vi "_2062021.vi"() -> ()   [LabVIEW 2020]
panel:
  in  "Stop Button":bool
  in  "LOAD":bool
  in  "SAVE":bool
  in  "Tremolo Enable":bool
  in  "Number of samples":i32=50000
  out "Tremolo Graph":dynamicdata(graph)
  in  "Tremelo Frequency":dbl(slide) scale=0.0..10.0
  in  "offset":dbl(slide) scale=0.0..10.0
  in  "Amplitude":dbl(slide) scale=0.0..10.0
  out "EQ Cluster":T1 {"Treble" scale=0.0..10.0; "Mid4" scale=0.0..10.0; "Mid3" scale=0.0..10.0; "Mid2" scale=0.0..10.0; "Mid1" scale=0.0..10.0; "Bass" scale=0.0..10.0}
  out "Output Graph":dynamicdata(graph)
  in  "Panning Enable":bool
  out "Equalizer Graph":dynamicdata(graph)
  in  "Enum":T2(ring)
  in  "Custom cluster":T1 {"Treble" scale=0.0..10.0; "Mid4" scale=0.0..10.0; "Mid3" scale=0.0..10.0; "Mid2" scale=0.0..10.0; "Mid1" scale=0.0..10.0; "Bass" scale=0.0..10.0}
  in  "EQ Enable":bool
  in  "Sampling rate":dbl=100000.0
  out "Panning Graph":dynamicdata(graph)
  in  "Panning Knob":dbl(knob) scale=-2.0..2.0
  in  "STOP":bool
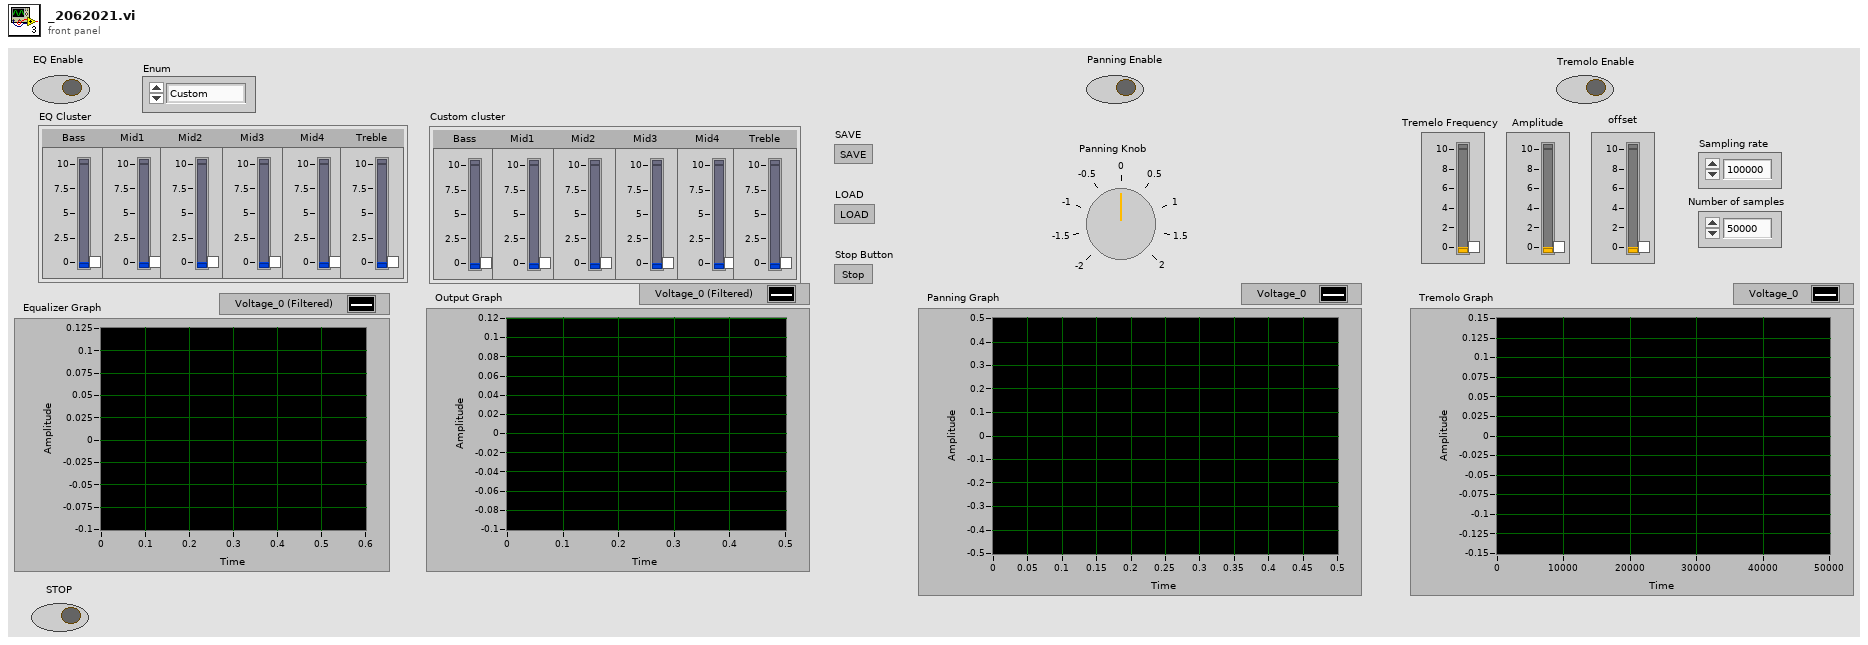
[diagram p1: front panel]
types:
  T1 = cluster{"Bass":dbl, "Mid1":dbl, "Mid2":dbl, "Mid3":dbl, "Mid4":dbl, "Treble":dbl}
  T2 = enum16{"Custom", "Flat", "Treble Boost", "Base Boost"}
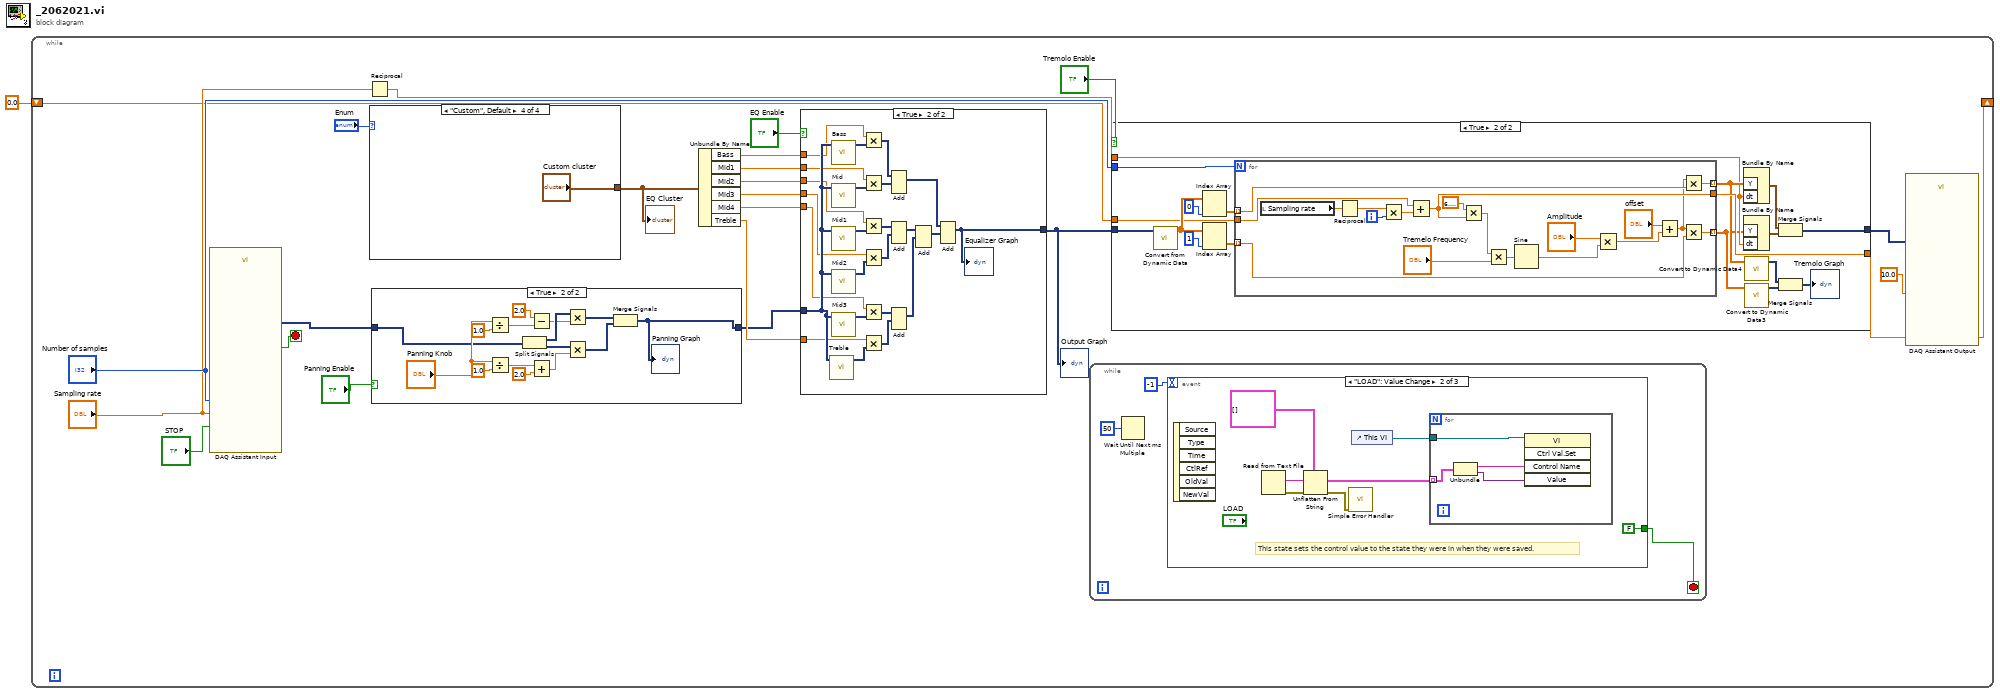
[diagram p0: block diagram]
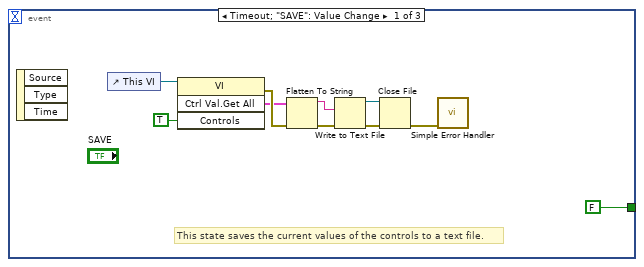
[diagram p2: hidden frame]
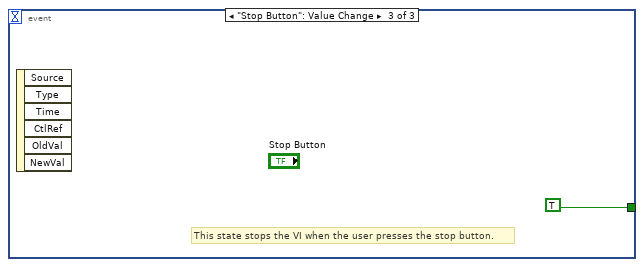
[diagram p3: hidden frame]
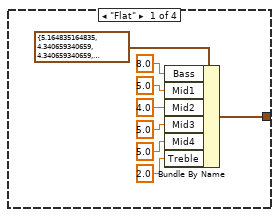
[diagram p6: hidden frame]
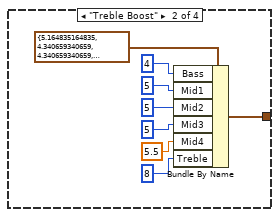
[diagram p7: hidden frame]
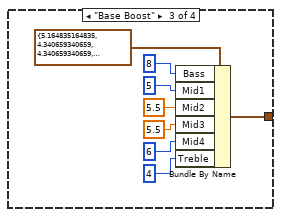
[diagram p8: hidden frame]
diagram:
  n1 = while {
    shift-right: [w10] -> _
    shift-left: 0.0 -> [w3]
    stop <- w23 stop-if-true
    n2 = call "DAQ Assistant Input"("rate"="Sampling rate", "number of samples"="Number of samples", "stop (F)"="STOP") -> ("data"=w15:dynamicdata, "stopped"=w23:bool)  [unwired: 13 in, 2 out]
    n3 = Reciprocal(x="Sampling rate") -> (1/x=w8:dbl)
    n4 = case shown="\"Custom\", Default" "Enum" {
      tunnel: [w105 w113 w121 "Custom cluster"] -> w11
      frame "Flat" {
        n5 = Bundle By Name(cluster=T1 {"Bass"=5.164835164835, "Mid1"=4.340659340659, "Mid2"=4.340659340659, "Mid3"=4.67032967033, "Mid4"=4.450549450549, "Treble"=5.3846153846149996} ("output cluster"), "Bass"=8.0, "Mid1"=5.0 ("Bass"), "Mid2"=4.0 ("Bass"), "Mid3"=5.0 ("Bass"), "Mid4"=5.0 ("Bass"), "Treble"=2.0 ("Bass")) -> (w105:T1)
      }
      frame "Treble Boost" {
        n6 = Bundle By Name(cluster=T1 {"Bass"=5.164835164835, "Mid1"=4.340659340659, "Mid2"=4.340659340659, "Mid3"=4.67032967033, "Mid4"=4.450549450549, "Treble"=5.3846153846149996} ("output cluster"), "Bass"=4, "Mid1"=5, "Mid2"=5, "Mid3"=5, "Mid4"=5.5, "Treble"=8) -> (w113:T1)
      }
      frame "Base Boost" {
        n7 = Bundle By Name(cluster=T1 {"Bass"=5.164835164835, "Mid1"=4.340659340659, "Mid2"=4.340659340659, "Mid3"=4.67032967033, "Mid4"=4.450549450549, "Treble"=5.3846153846149996} ("input cluster"), "Bass"=8, "Mid1"=5, "Mid2"=5.5, "Mid3"=5.5, "Mid4"=6, "Treble"=4) -> (w121:T1)
      }
      frame "Custom", Default {
      }
    }
    "EQ Cluster" <- w11
    n8 = case shown="True" "Panning Enable" {
      tunnel: w15 -> [w89 w91]
      tunnel: [w89 w90] -> w14
      frame False {
      }
      frame True {
        n9 = Divide(x="Panning Knob", y=1.0) -> (x/y=w102:dbl)
        n10 = Divide(x="Panning Knob", y=1.0) -> (x/y=w95:dbl)
        n11 = Split Signals(w91) -> (w104:dynamicdata, w94:dynamicdata)  [unwired: 2 in]
        n12 = Subtract(x=2.0, y=w102) -> (x-y=w100:dbl)
        n13 = Add(x=w95, y=2.0 ("x")) -> (x+y=w97:dbl)
        n14 = Multiply(x=w104, y=w100) -> (x*y=w93:dynamicdata)
        n15 = Multiply(x=w94, y=w97) -> (x*y=w92:dynamicdata)
        n16 = Merge Signals(w93, w92) -> (w90:dynamicdata)
        "Panning Graph" <- w90
      }
    }
    n17 = Unbundle By Name(w11) -> ("Bass"=w22:dbl, "Mid1"=w21:dbl, "Mid2"=w20:dbl, "Mid3"=w19:dbl, "Mid4"=w18:dbl, "Treble"=w17:dbl)
    n18 = case shown="True" "EQ Enable" {
      tunnel: w14 -> [w130 w154]
      tunnel: w22 -> [_ w147]
      tunnel: w21 -> [_ w146]
      tunnel: w20 -> [_ w145]
      tunnel: w19 -> [_ w144]
      tunnel: w18 -> [_ w143]
      tunnel: w17 -> [_ w142]
      tunnel: [w130 w132] -> w9
      frame False {
      }
      frame True {
        n19 = call "Treble"("Signal"=w154) -> ("Filtered Signal"=w148:dynamicdata)  [unwired: 9 in, 1 out]
        n20 = call "Bass"("Signal"=w154) -> ("Filtered Signal"=w153:dynamicdata)  [unwired: 9 in, 1 out]
        n21 = call "Mid"("Signal"=w154) -> ("Filtered Signal"=w152:dynamicdata)  [unwired: 9 in, 1 out]
        n22 = call "Mid1"("Signal"=w154) -> ("Filtered Signal"=w151:dynamicdata)  [unwired: 9 in, 1 out]
        n23 = call "Mid2"("Signal"=w154) -> ("Filtered Signal"=w150:dynamicdata)  [unwired: 9 in, 1 out]
        n24 = call "Mid3"("Signal"=w154) -> ("Filtered Signal"=w149:dynamicdata)  [unwired: 9 in, 1 out]
        n25 = Multiply(x=w147, y=w153) -> (x*y=w141:dynamicdata)
        n26 = Multiply(x=w146, y=w152) -> (x*y=w140:dynamicdata)
        n27 = Multiply(x=w145, y=w151) -> (x*y=w139:dynamicdata)
        n28 = Multiply(x=w144, y=w150) -> (x*y=w138:dynamicdata)
        n29 = Multiply(x=w143, y=w149) -> (x*y=w137:dynamicdata)
        n30 = Multiply(x=w142, y=w148) -> (x*y=w136:dynamicdata)
        n31 = Add(1:w140, 2:w141) -> (0:w133:dynamicdata)  [unwired: 1 in, 1 out]
        n32 = Add(1:w138, 2:w139) -> (0:w135:dynamicdata)  [unwired: 1 in, 1 out]
        n33 = Add(1:w136, 2:w137) -> (0:w131:dynamicdata)  [unwired: 1 in, 1 out]
        n34 = Add(1:w131, 2:w135) -> (0:w134:dynamicdata)  [unwired: 1 in, 1 out]
        n35 = Add(1:w134, 2:w133) -> (0:w132:dynamicdata)  [unwired: 1 in, 1 out]
        "Equalizer Graph" <- w132
      }
    }
    "Output Graph" <- w9
    n36 = while {
      stop <- w27 stop-if-true
      n37 = Wait Until Next ms Multiple(millisecond multiple=u32 50) -> ()  [unwired: 1 out]
      n38 = event shown="[1] \"LOAD\": Value Change" {
        selector: _ -> [_ _ _]
        dyn-events: _ -> [_ _ _]
        timeout: -1 -> [_ _ _]
        tunnel: [FALSE FALSE TRUE] -> w27
        event Timeout; "SAVE": Value Change {
          # "This state saves the current values of the controls to a text file."
          n39 = event-data() -> ()  [unwired: 1 in, 3 out]
          n40 = control-ref of="This VI"() -> (w37:refnum<vi>)
          n41 = invoke class="VI" method="Ctrl Val.Get All"(reference=w37, "Controls"=TRUE) -> (error out=w33:errorcluster, "Get All Control Values Variant"=w32:cluster{"Name":string, "Variant Data":variant}[])  [unwired: 2 in, 2 out]
          n42 = Flatten To String(anything=w32, error in (no error)=w33) -> (data string=w34:string, error out=w35:errorcluster)  [unwired: 2 in, 1 out]
          n43 = Write to Text File(text=w34, error in=w35) -> (refnum out=w30:refnum<file>, error out=w31:errorcluster)  [unwired: 2 in, 1 out]
          n44 = Close File(refnum=w30, error in=w31) -> (error out=w29:errorcluster)  [unwired: 1 out]
          n45 = call <vilib>:"Simple Error Handler.vi"("error in (no error)"=w29) -> ()  [unwired: 4 in, 5 out]
        }
        event "LOAD": Value Change {
          # "This state sets the control value to the state they were in when they were saved."
          n46 = event-data() -> ()  [unwired: 1 in, 6 out]
          n47 = Read from Text File() -> (text=w42:string, error out=w43:errorcluster)  [unwired: 4 in, 2 out]
          n48 = Unflatten From String(type=cluster{string, variant}[] [], binary string=w42, error in (no error)=w43) -> (value=w40:cluster{string, variant}[], error out=w38:errorcluster)  [unwired: 2 in, 1 out]
          n49 = call <vilib>:"Simple Error Handler.vi"("error in (no error)"=w38) -> ()  [unwired: 4 in, 5 out]
          n50 = control-ref of="This VI"() -> (w41:refnum<vi>)
          n51 = for {
            tunnel: w41 -> [w48]
            tunnel: w40 -> [w47] mode=indexing
            n52 = Unbundle(w47) -> (w45:string, w46:variant)
            n53 = invoke class="VI" method="Ctrl Val.Set"(reference=w48, "Control Name"=w45, "Value"=w46) -> ()  [unwired: 2 in, 5 out]
          }
        }
        event "Stop Button": Value Change {
          # "This state stops the VI when the user presses the stop button."
          n54 = event-data() -> ()  [unwired: 1 in, 6 out]
        }
      }
    }
    n55 = case shown="True" "Tremolo Enable" {
      tunnel: [w50 w64] -> w10
      tunnel: w9 -> [w51 w60]
      tunnel: w8 -> [_ w58]
      tunnel: [w51 w54] -> w7
      tunnel: "Number of samples" -> [_ w53]
      tunnel: w3 -> [w50 w52]
      frame False {
      }
      frame True {
        n56 = call "Convert from Dynamic Data"("Dynamic Data Type"=w60) -> ("Array"=w68:dbl[][])  [unwired: 3 in]
        n57 = Index Array(array=w68, index (col)=0 ("disabled index (col)")) -> (element=w66:dbl[])  [unwired: 1 in]
        n58 = Index Array(array=w68, index (col)=1 ("disabled index (col)")) -> (element=w65:dbl[])  [unwired: 1 in]
        n59 = for {
          N: w53 -> [_]
          tunnel: w66 -> [w75] mode=indexing
          tunnel: w65 -> [w74] mode=indexing
          tunnel: [w83] -> w64
          tunnel: w52 -> [w86]
          tunnel: [w72] -> w59 mode=indexing
          tunnel: [w71] -> w57 mode=indexing
          i -> [w87]
          n60 = local read "Sampling rate"() -> (w70:dbl)
          n61 = Reciprocal(x=w70) -> (1/x=w88:dbl)
          n62 = Multiply(x=w88, y=w87) -> (x*y=w85:dbl)
          n63 = Add(x=w86, y=w85) -> (x+y=w83:dbl)
          n64 = Multiply(x=6.283185307179586, y=w83) -> (x*y=w78:dbl)
          n65 = Multiply(x=w78, y="Tremelo Frequency") -> (x*y=w77:dbl)
          n66 = Sine(x=w77) -> (sin(x)=w82:dbl)
          n67 = Multiply(x="Amplitude", y=w82) -> (x*y=w80:dbl)
          n68 = Add(x="offset", y=w80) -> (x+y=w73:dbl)
          n69 = Multiply(x=w73, y=w75) -> (x*y=w72:dbl)
          n70 = Multiply(x=w73, y=w74) -> (x*y=w71:dbl)
        }
        n71 = Bundle By Name("Y"=w59, "dt"=w58) -> (w55:waveform(dbl))  [unwired: 1 in]
        n72 = Bundle By Name("Y"=w57, "dt"=w58) -> (w56:waveform(dbl))  [unwired: 1 in]
        n73 = call "Convert to Dynamic Data4"("Array"=w59) -> ("Dynamic Data Type"=w63:dynamicdata)  [unwired: 3 in]
        n74 = call "Convert to Dynamic Data3"("Array"=w57) -> ("Dynamic Data Type"=w62:dynamicdata)  [unwired: 3 in]
        n75 = Merge Signals(w55, w56) -> (w54:dynamicdata)
        n76 = Merge Signals(w63, w62) -> (→"Tremolo Graph":dynamicdata)
      }
    }
    n77 = call "DAQ Assistant Output"("data"=w7, "timeout (s)"=10.0) -> ()  [unwired: 15 in, 3 out]
  }
